vi "ConvertShiftsToScanCoordinates.vi"(9 "PixelToScanCoordConvFactors":T2={"Dx_drow"=1.0, "Dy_drow"=1.0, "Dz_drow"=1.0, "Dx_dcol"=1.0, "Dy_dcol"=1.0, "Dz_dcol"=1.0} {"Dz_dcol" format="%0.2f"; "Dy_dcol" format="%0.2f"; "Dx_dcol" format="%0.2f"; "Dz_drow" format="%0.2f"; "Dy_drow" format="%0.2f"; "Dx_drow" format="%0.2f"}, 10 "Col Shift Array":dbl[](array[numeric]), 11 "Row Shift Array":dbl[](array[numeric])) -> (3 "Motion":T1)   [LabVIEW 2014]
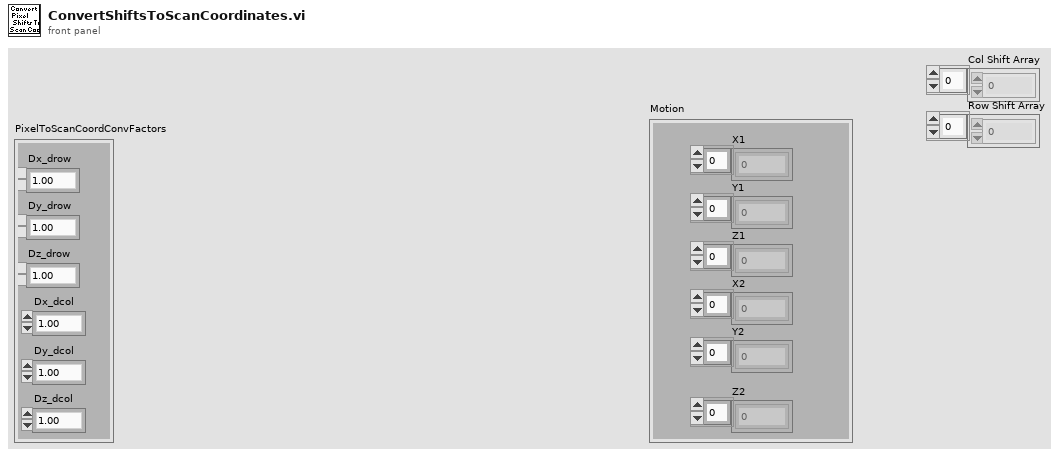
[diagram p1: front panel]
types:
  T1 = cluster{"X1":dbl[], "Y1":dbl[], "Z1":dbl[], "X2":dbl[], "Y2":dbl[], "Z2":dbl[]}
  T2 = cluster{"Dx_drow":dbl, "Dy_drow":dbl, "Dz_drow":dbl, "Dx_dcol":dbl, "Dy_dcol":dbl, "Dz_dcol":dbl}
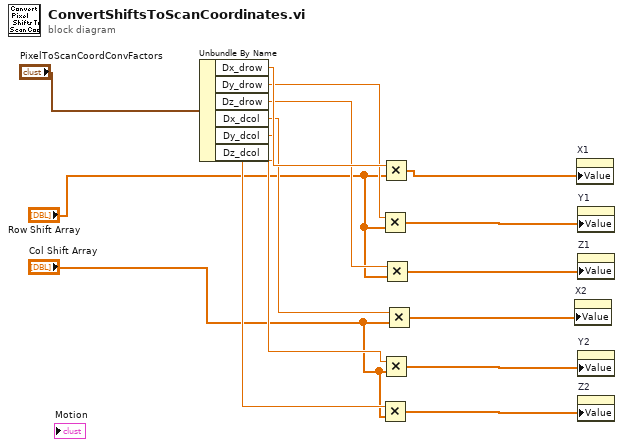
[diagram p0: block diagram]
diagram:
  n1 = Unbundle By Name("PixelToScanCoordConvFactors") -> ("Dx_drow"=w14:dbl, "Dy_drow"=w13:dbl, "Dz_drow"=w12:dbl, "Dx_dcol"=w11:dbl, "Dy_dcol"=w10:dbl, "Dz_dcol"=w9:dbl)
  n2 = Multiply(x=w13, y="Row Shift Array") -> (x*y=w6:dbl[])
  n3 = Multiply(x=w9, y="Col Shift Array") -> (x*y=w1:dbl[])
  n4 = Multiply(x=w14, y="Row Shift Array") -> (x*y=w7:dbl[])
  n5 = Multiply(x=w10, y="Col Shift Array") -> (x*y=w2:dbl[])
  n6 = Multiply(x=w12, y="Row Shift Array") -> (x*y=w5:dbl[])
  n7 = Multiply(x=w11, y="Col Shift Array") -> (x*y=w3:dbl[])
  n8 = property on="X2" class="Arr (strict)"("Value"=w3) -> ()  [unwired: 2 in, 2 out]
  n9 = property on="X1" class="Arr (strict)"("Value"=w7) -> ()  [unwired: 2 in, 2 out]
  n10 = property on="Y1" class="Arr (strict)"("Value"=w6) -> ()  [unwired: 2 in, 2 out]
  n11 = property on="Z1" class="Arr (strict)"("Value"=w5) -> ()  [unwired: 2 in, 2 out]
  n12 = property on="Y2" class="Arr (strict)"("Value"=w2) -> ()  [unwired: 2 in, 2 out]
  n13 = property on="Z2" class="Arr (strict)"("Value"=w1) -> ()  [unwired: 2 in, 2 out]
